vi "Initialize.vi"(8 "error in":errorcluster, 10 "parameters":variant, 11 "node in":refnum<class "module editor node.lvclass">) -> (0 "error out":errorcluster, 2 "summary":T2[](array[typedef]), 3 "data value reference":T1)   [LabVIEW 2013, in "PL Framework Configuration Tool.lvlib" / "module editor node.lvclass"]
doc: "Initializes the data of a node to its default state.\nThe object is not created inside of this VI, because it is created from a File depending on user selection."
uses:
  module editor node.lvclass
  <vilib>/NI/CEF/CEF_TreeControl/Node/Summary.ctl
  <vilib>/NI/CEF/CEF_TreeControl/Node/NodeRef.ctl
  <vilib>/NI/CEF/CEF_TreeControl/Node/NISE_CEF_Node.lvclass
  TBM Configuration Node/TBM Configuration Node.lvclass
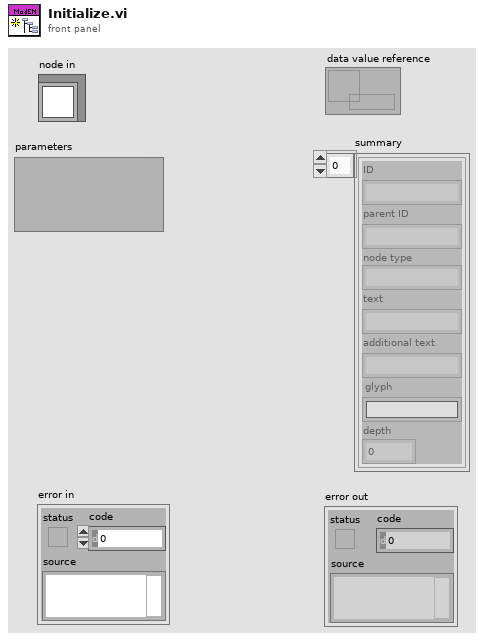
[diagram p1: front panel]
types:
  T1 = typedef "NISE_CEF_Node.lvclass/NodeRef.ctl" = refnum<data-value>
  T2 = typedef "NISE_CEF_Node.lvclass/Summary.ctl" = cluster{"ID":string, "parent ID":string, "node type":string, "text":string, "additional text":string, "glyph":string, "depth":i32}
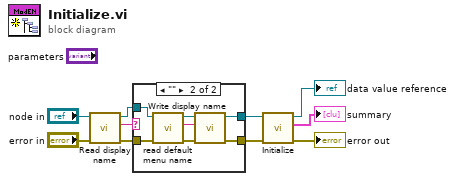
[diagram p0: block diagram]
diagram:
  n1 = call "Read display name.vi"("error in"="error in", "module editor node in"="node in") -> ("error out"=w3:errorcluster, "display name"=w4:string, "module editor node out"=w5:refnum<class "module editor node.lvclass">)  [unwired: 7 in]
  n2 = case shown="\"\"" w4 {
    tunnel: [w11 w19] -> w9
    tunnel: [w12 w18] -> w8
    tunnel: w3 -> [w11 w16]
    tunnel: w5 -> [w12 w17]
    frame Default {
    }
    frame "" {
      n3 = call-dynamic "read default menu name.vi"("error in"=w16, "module editor node in"=w17) -> ("error out"=w15:errorcluster, "default menu name"=w14:string, "module editor node out"=w13:refnum<class "module editor node.lvclass">)  [unwired: 7 in]
      n4 = call "Write display name.vi"("error in"=w15, "display name"=w14, "module editor node in"=w13) -> ("error out"=w19:errorcluster, "module editor node out"=w18:refnum<class "module editor node.lvclass">)  [unwired: 7 in]
    }
  }
  n5 = call-parent "Initialize.vi"("error in"=w9, "node in"=w8) -> ("error out"=→"error out":errorcluster, "summary"=→"summary":T2[], "data value reference"=→"data value reference":T1)  [unwired: 7 in]
